vi "Evaluate Captured Waveforms 2.vi"(8 "error in":errorcluster, 11 "Original Live Graph Plotter":refnum<class "Live Graph Plotter.lvclass">) -> (0 "error out":errorcluster, 3 "Response Passed?":bool)   [LabVIEW 2025]
uses:
  Live Graph Plotter/Live Graph Plotter.lvclass
panel:
  out "Post Processed Waveforms":T1(graph)
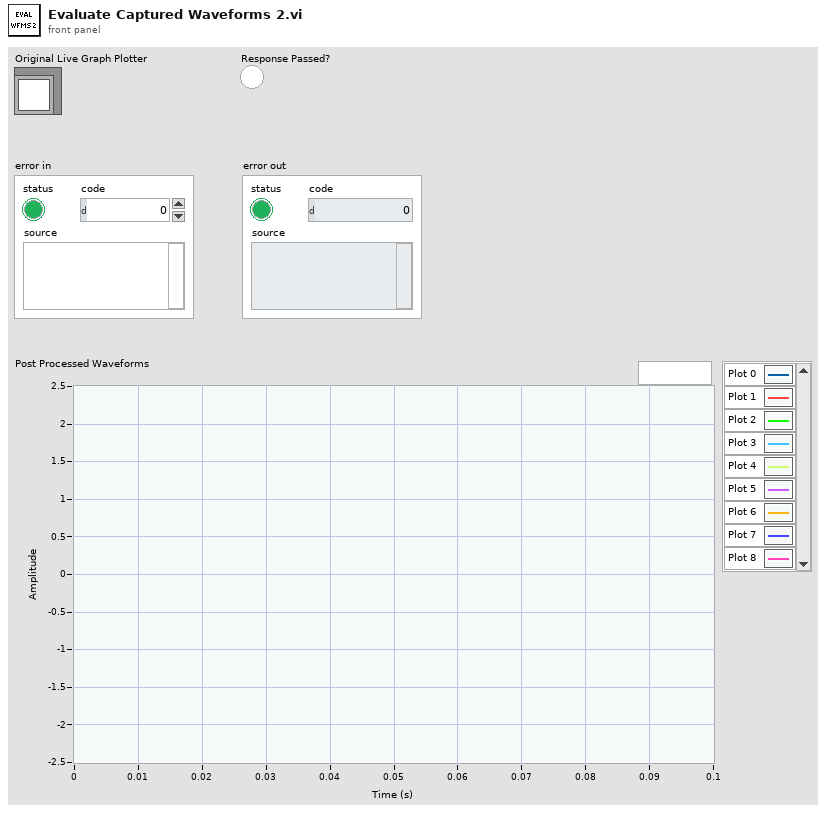
[diagram p1: front panel]
types:
  T1 = cluster{"relativeInitialX":dbl, "xIncrement":dbl, "wfm":dbl[]}[]
  T2 = cluster{"Record Start Index (0)":i32, "Record Length (-1)":i32, "Channel List (All)":string}
  T3 = cluster{"Channel Name":string, "relativeInitialX":dbl, "xIncrement":dbl, "Waveforms":cluster{"wfm":dbl[]}[]}[]
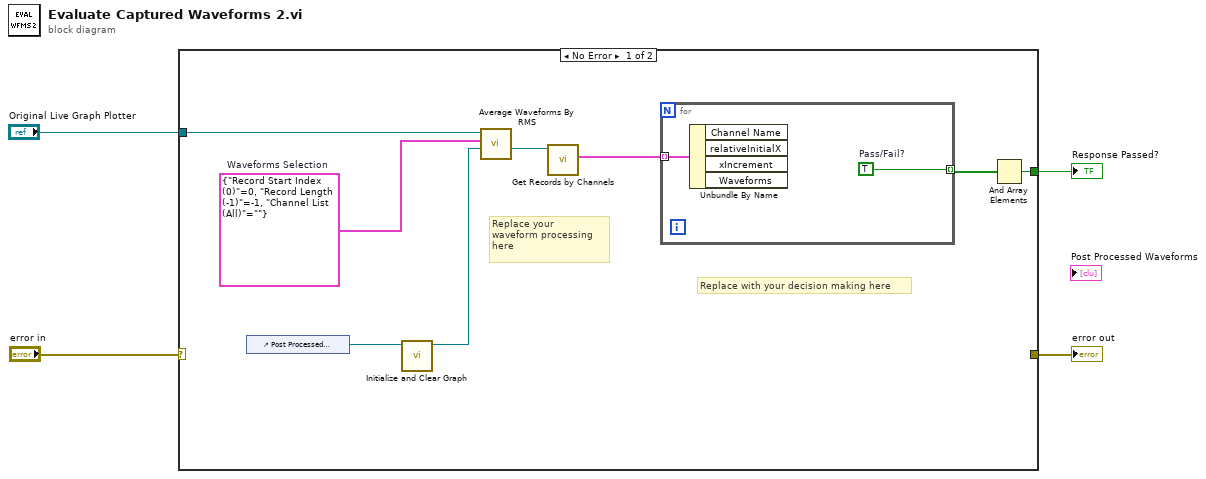
[diagram p0: block diagram]
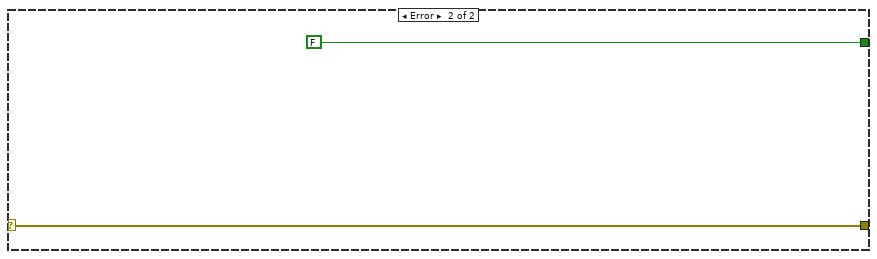
[diagram p2: hidden frame]
diagram:
  n1 = case shown="No Error" "error in" {
    selector: "error in" -> [_ w16]
    tunnel: [w12 FALSE] -> w4
    tunnel: [_ w16] -> w2
    tunnel: "Original Live Graph Plotter" -> [w10 _]
    frame No Error {
      w5 = T2 {"Record Start Index (0)"=0, "Record Length (-1)"=-1, "Channel List (All)"=""}  # Waveforms Selection
      # "Replace with your decision making here"
      # "Replace your\nwaveform processing \nhere"
      n2 = control-ref of="Post Processed Waveforms"() -> (w9:refnum<vi>)
      n3 = call "Initialize and Clear Graph.vi"("WaveformGraph Ref"=w9) -> ("Live Graph Plotter out"=w8:refnum<class "Live Graph Plotter.lvclass">)  [unwired: 9 in, 1 out]
      n4 = call "Average Waveforms By RMS.vi"("Result Live Graph Plotter in"=w8, "Waveforms Selection"=w5, "Original Live Graph Plotter in"=w10) -> ("Result Live Graph Plotter out"=w7:refnum<class "Live Graph Plotter.lvclass">)  [unwired: 7 in, 1 out]
      n5 = call "Get Records by Channels.vi"("Live Graph Plotter in"=w7) -> ("Records By Channels"=w6:T3)  [unwired: 7 in, 3 out]
      n6 = for {
        tunnel: [w14] -> w11 mode=indexing
        tunnel: w6 -> [w13] mode=indexing
        w14 = TRUE  # Pass/Fail?
        n7 = Unbundle By Name(w13) -> ()  [unwired: 4 out]
      }
      n8 = And Array Elements(Boolean array=w11) -> (logical AND=w12:bool)
    }
    frame Error {
    }
  }
  "Response Passed?" <- w4
  "error out" <- w2
